vi "monochromatorCommandSetSteps.vi"(8 "error in":errorcluster, 10 "step":i32, 11 "monochromator":refnum<k24>) -> (0 "error out":errorcluster, 2 "wavelength":dbl, 3 "monochromator":refnum<k24>)   [LabVIEW 2009]
doc: "Get shutter status\nFALSE = Shutter is CLOSED\nTRUE = Shutter is OPEN"
uses:
  C:/Users/anderson.chen/Desktop/Software Development/Cornerstone Series API (LV9)/Cornerstone DLL/Cornerstone.dll
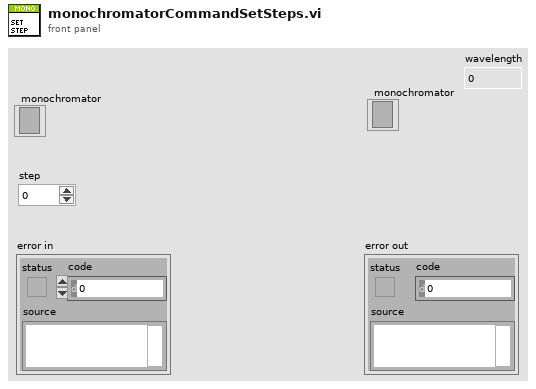
[diagram p1: front panel]
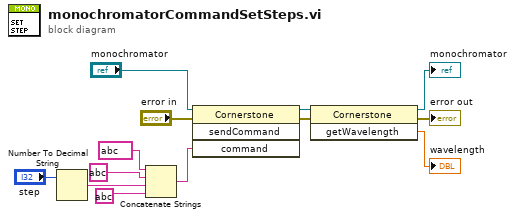
[diagram p0: block diagram]
diagram:
  n1 = Number To Decimal String(number="step") -> (decimal integer string=w3:string)  [unwired: 1 in]
  n2 = Concatenate Strings(string ? ("command in"), string ?, w3, string ?) -> (w7:string)
  n3 = invoke class="Cornerstone" method="sendCommand"(reference="monochromator", error in="error in", "command"=w7) -> (reference out=w2:refnum<k24>, error out=w1:errorcluster)  [unwired: 1 in, 2 out]
  n4 = invoke class="Cornerstone" method="getWavelength"(reference=w2, error in=w1) -> (reference out=→"monochromator":refnum<k24>, error out=→"error out":errorcluster, "getWavelength"=→"wavelength":dbl)  [unwired: 1 in]
